vi "Change RepRate.vi"(0 "nCRD in":refnum<class "nCRD.lvclass">, 5 "error in":errorcluster) -> (14 "nCRD out":refnum<class "nCRD.lvclass">, 19 "error out":errorcluster)   [LabVIEW 2015, in "nCRD.lvclass"]
uses:
  nCRD.lvclass
  nCRD.lvclass/nCRD.ctl
  <vilib>/Utility/error.llb/Error Cluster From Error Code.vi
  <vilib>/rvi/errors/niLvFpgaAdjustHostInterfaceError.vi
  <vilib>/rvi/interface/nirviReadWriteControl/nirviReadWriteControl.xnode
  FPGA Ref.ctl
  FPGA Bitfiles/NickIO.lvbitx
  <vilib>/rvi/interface/nirviMethod/nirviMethod.xnode
  NiFpgaLv.dll
  <vilib>/FPGAPlugInAG/cRIO-9081/niLvFpga_ReadFifo_cRIO-9081.vi
  <vilib>/rvi/errors/niLvFpgaMergeErrorWithErrorCode.vi
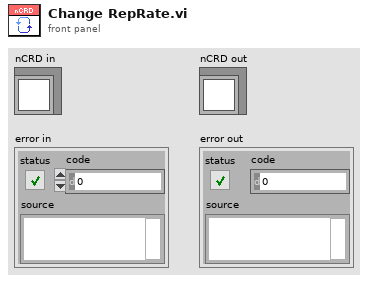
[diagram p1: front panel]
types:
  T1 = typedef "FPGA Ref.ctl" = refnum<k20>
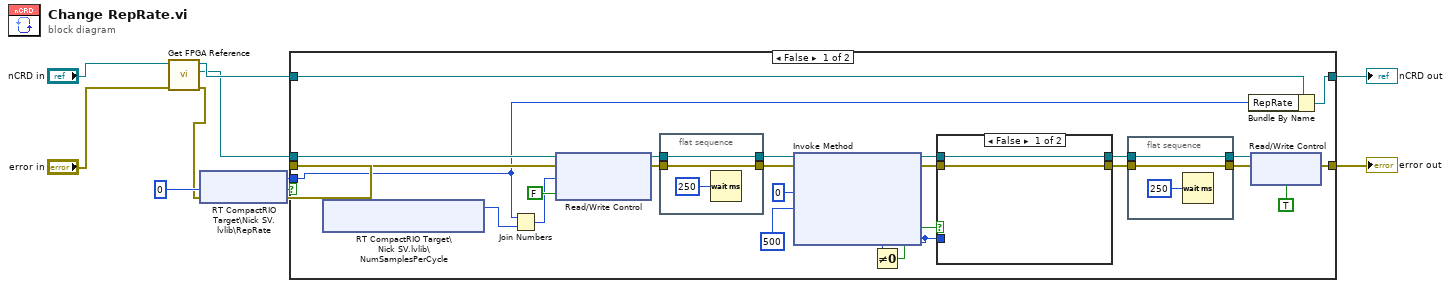
[diagram p0: block diagram]
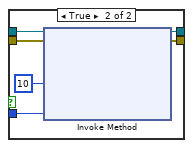
[diagram p2: hidden frame]
diagram:
  n1 = call "Get FPGA Reference.vi"("error in (no error)"="error in", "nCRD in"="nCRD in") -> ("error out"=w2:errorcluster, "Accessors:FPGA Ref"=w3:T1, "nCRD Out"=w4:refnum<class "nCRD.lvclass">)  [unwired: 7 in]
  n2 = shared-variable "RT CompactRIO Target\\Nick SV.lvlib\\RepRate"(error in=w2, 0 ("ms timeout (0)")) -> (w9:u16, error out=w1:errorcluster, w8:bool)
  n3 = case shown="False" w8 {
    tunnel: [w35 w51] -> w10
    tunnel: w4 -> [w34 w51]
    tunnel: w3 -> [w33 _]
    tunnel: w9 -> [w13 _]
    tunnel: [w32 w50] -> w11
    tunnel: w1 -> [w31 w50]
    frame False {
      n4 = shared-variable "RT CompactRIO Target\\Nick SV.lvlib\\NumSamplesPerCycle"() -> (w14:u16)  [unwired: 2 in, 2 out]
      n5 = Join Numbers(hi=w13, lo=w14) -> ((hi.lo)=w12:u32)
      n6 = xnode "Read/Write Control"("FPGA VI Reference In"=w33, "error in"=w31, "CRDSampData"=w12, "Transmit?"=FALSE) -> ("FPGA VI Reference Out"=w19:T1, "error out"=w29:errorcluster)
      n7 = flat-sequence {
        tunnel: w29 -> [w45]
        tunnel: [w45] -> w27
        tunnel: w19 -> [w44]
        tunnel: [w44] -> w18
        frame #0 {
          n8 = Wait (ms)(milliseconds to wait=u32 250) -> ()  [unwired: 1 out]
        }
      }
      n9 = xnode "Invoke Method"("FPGA VI Reference In"=w18, "error in"=w27, "Number of Elements"=u32 0, "Timeout (ms)"=500) -> ("FPGA VI Reference Out"=w25:T1, "error out"=w26:errorcluster, "Elements Remaining"=w16:u32)  [unwired: 1 out]
      n10 = Not Equal To 0?(x=w16) -> (x != 0?=w15:bool)
      n11 = case shown="False" w15 {
        tunnel: w26 -> [w36 w43]
        tunnel: w25 -> [w37 w42]
        tunnel: [w36 w41] -> w23
        tunnel: w16 -> [_ w40]
        tunnel: [w37 w38] -> w21
        frame False {
        }
        frame True {
          n12 = xnode "Invoke Method"("FPGA VI Reference In"=w42, "error in"=w43, "Number of Elements"=w40, "Timeout (ms)"=10) -> ("FPGA VI Reference Out"=w38:T1, "error out"=w41:errorcluster)  [unwired: 2 out]
        }
      }
      n13 = flat-sequence {
        tunnel: w23 -> [w48]
        tunnel: [w48] -> w24
        tunnel: w21 -> [w47]
        tunnel: [w47] -> w20
        frame #0 {
          n14 = Wait (ms)(milliseconds to wait=u32 250) -> ()  [unwired: 1 out]
        }
      }
      n15 = Bundle By Name(cluster=w34, "RepRate"=w13) -> (w35:refnum<class "nCRD.lvclass">)
      n16 = xnode "Read/Write Control"("FPGA VI Reference In"=w20, "error in"=w24, "Transmit?"=TRUE) -> ("error out"=w32:errorcluster)  [unwired: 1 out]
    }
    frame True {
    }
  }
  "error out" <- w11
  "nCRD out" <- w10
